vi "save_files.vi"(4 "List Parameter Fit":dbl[][](array[numeric]), 5 "data_test":T1, 6 "Param Calibrazione":T2, 8 "error in (no error)":errorcluster, 10 "List ROI":dbl[][](array[numeric]), 11 "Table in":refnum<vi>) -> (0 "error out":errorcluster)   [LabVIEW 2023]
uses:
  control/param_calibrazione.ctl
  control/global name path.vi
  <vilib>/Utility/file.llb/Write Delimited Spreadsheet (DBL).vi
  <vilib>/Utility/file.llb/Write Delimited Spreadsheet (string).vi
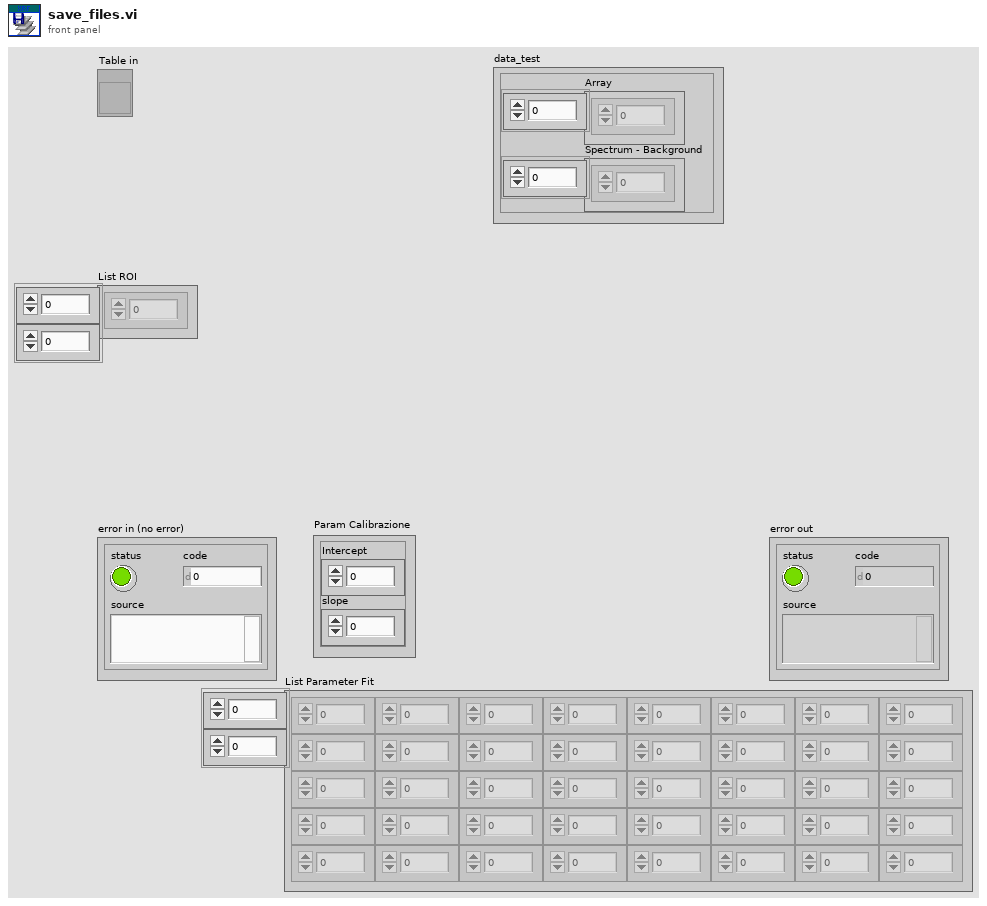
[diagram p1: front panel]
types:
  T1 = cluster{"Array":dbl[], "Spectrum - Background":dbl[]}
  T2 = typedef "param_calibrazione.ctl" = cluster{"Intercept":dbl, "slope":dbl}
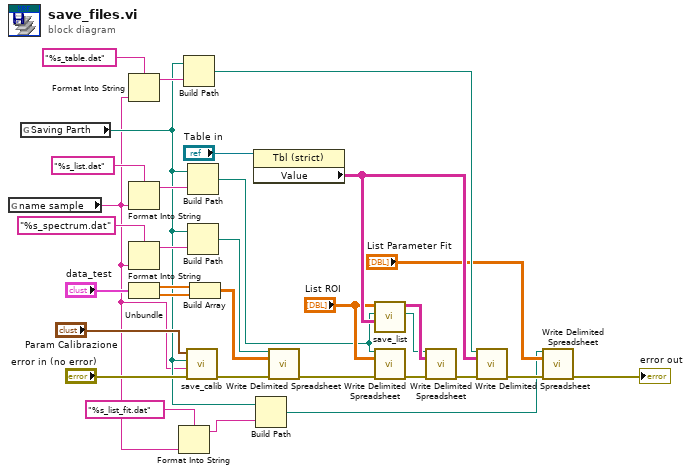
[diagram p0: block diagram]
diagram:
  n1 = global read "global name path.vi" "name sample"() -> (w1:string)
  n2 = global read "global name path.vi" "Saving Parth"() -> (w2:path)
  n3 = Format Into String(format string="%s_table.dat", w1) -> (resulting string=w19:string)  [unwired: 2 in, 1 out]
  n4 = Format Into String(format string="%s_list.dat", w1) -> (resulting string=w18:string)  [unwired: 2 in, 1 out]
  n5 = Format Into String(format string="%s_spectrum.dat", w1) -> (resulting string=w17:string)  [unwired: 2 in, 1 out]
  n6 = Unbundle("data_test") -> ("Array"=w11:dbl[], "Spectrum - Background"=w12:dbl[])
  n7 = Format Into String(format string="%s_list_fit.dat", w1) -> (resulting string=w7:string)  [unwired: 2 in, 1 out]
  n8 = Build Path(base path=w2, name or relative path=w19) -> (appended path=w21:path)
  n9 = call "save_calib.vi"("error in (no error)"="error in (no error)", "name sample"=w1, "Save Path"=w2, "Param. Calib"="Param Calibrazione") -> ("error out"=w31:errorcluster)  [unwired: 7 in]
  n10 = Build Path(base path=w2, name or relative path=w18) -> (appended path=w23:path)
  n11 = Build Path(base path=w2, name or relative path=w17) -> (appended path=w20:path)
  n12 = Build Array(w11, w12) -> (w13:dbl[][])
  n13 = property on="Property Node" class="Tbl (strict)"(reference="Table in") -> ("Value"=w29:string[][])  [unwired: 1 in, 2 out]
  n14 = Build Path(base path=w2, name or relative path=w7) -> (appended path=w4:path)
  n15 = call-poly <vilib>:"Write Delimited Spreadsheet.vi"("file path (dialog if empty)"=w20, "2D data"=w13, "error in (no error)"=w31) -> ("error out"=w22:errorcluster)  [unwired: 11 in, 1 out]
  n16 = call "save_list.vi"("Elements Selected"=w29, "list path in"=w23, "List ROI in"="List ROI") -> ("list path out"=w25:path, "list array"=w26:string[][])  [unwired: 7 in]
  n17 = call-poly <vilib>:"Write Delimited Spreadsheet.vi"("file path (dialog if empty)"=w23, "2D data"="List ROI", "error in (no error)"=w22) -> ("error out"=w27:errorcluster)  [unwired: 11 in, 1 out]
  n18 = call-poly <vilib>:"Write Delimited Spreadsheet.vi"("file path (dialog if empty)"=w25, "2D data"=w26, "error in (no error)"=w27) -> ("error out"=w28:errorcluster)  [unwired: 11 in, 1 out]
  n19 = call-poly <vilib>:"Write Delimited Spreadsheet.vi"("file path (dialog if empty)"=w21, "2D data"=w29, "error in (no error)"=w28) -> ("error out"=w6:errorcluster)  [unwired: 11 in, 1 out]
  n20 = call-poly <vilib>:"Write Delimited Spreadsheet.vi"("file path (dialog if empty)"=w4, "2D data"="List Parameter Fit", "error in (no error)"=w6) -> ("error out"=→"error out":errorcluster)  [unwired: 11 in, 1 out]
